vi "Lake Shore 335.vi"(6 "Setpoint":dbl format="%.4f", 7 "VISA resource name":refnum<visa-resource-name>, 8 "Range":u16(ring) items=["Off", "Low (On)", "Medium", "High"], 9 "Rate (D) (X.X %)":dbl=120.0 format="%.1f", 10 "Reset (I) (XX.X)":dbl=20.0 format="%.1f", 11 "Gain (P) (XX.X)":dbl=50.0 format="%.1f") -> (0 "Setpoint":dbl format="%.4f", 1 "Heater 1 (%)":dbl format="%.1f", 2 "Input B":dbl, 3 "Input A":dbl)   [LabVIEW 2012]
doc: "This example VI demonstrates the proper use of the Sensor Data (Multiple Readings) VI. This VI reads and returns multiple sensor readings from the instrument. Control over interval between readings is also provided."
uses:
  <instrlib>/Lake Shore 335/Public/Data/Sensor Data (Single Reading).vi
  <instrlib>/Lake Shore 335/Lake Shore 335.lvlib
panel:
  in  "Manual Output":dbl format="%.2f"
  out "Rate (D)":dbl format="%.1f"
  out "Reset (I)":dbl=20.0 format="%.1f"
  out "Gain (P)":dbl=50.0 format="%.1f"
  in  "Unit":u16(ring)=1 items=["Kelvin", "Celcius", "Sensor"]
  in  "Unit":u16(ring)=1 items=["Kelvin", "Celcius", "Sensor"]
  in  "stop":bool
  in  "Serial Configuration":T1={"Baud Rate"=57600, "Parity"=1, "Data Bits"=7, "Stop Bits"=10, "Flow Control"=0} {"Flow Control" items=["None", "XON/XOFF", "RTS/CTS", "XON/XOFF & RTS/CTS", "DTR/DSR", "XON/XOFF & DTR/DSR"]; "Stop Bits" items=["1.0"=10, "1.5"=15, "2.0"=20]; "Data Bits" items=["7"=7, "8"=8]; "Parity" items=["None", "Odd", "Even", "Mark", "Space"]; "Baud Rate" items=["300"=300, "600"=600, "1200"=1200, "2400"=2400, "4800"=4800, "9600"=9600, "19200"=19200, "38400"=38400, "57600"=57600]}
  # "Setpoint Configuration"
  # "Sensor Data"
  # "PID Configuration"
  # "Connection Settings"
  # "PID Controlling on Input A"
  # "PID Controlling on Input A"
  # "PID Read Oud (Check)"
  # "Heater Output"
  # "Setpoint Read Out (Check)"
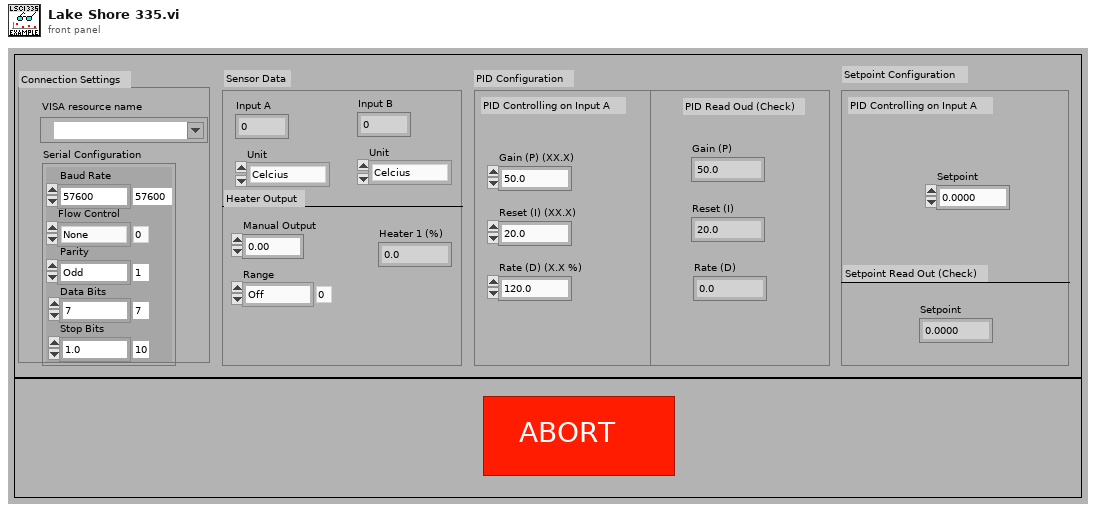
[diagram p1: front panel]
types:
  T1 = cluster{"Baud Rate":u32, "Parity":u16, "Data Bits":u16, "Stop Bits":u16, "Flow Control":u16}
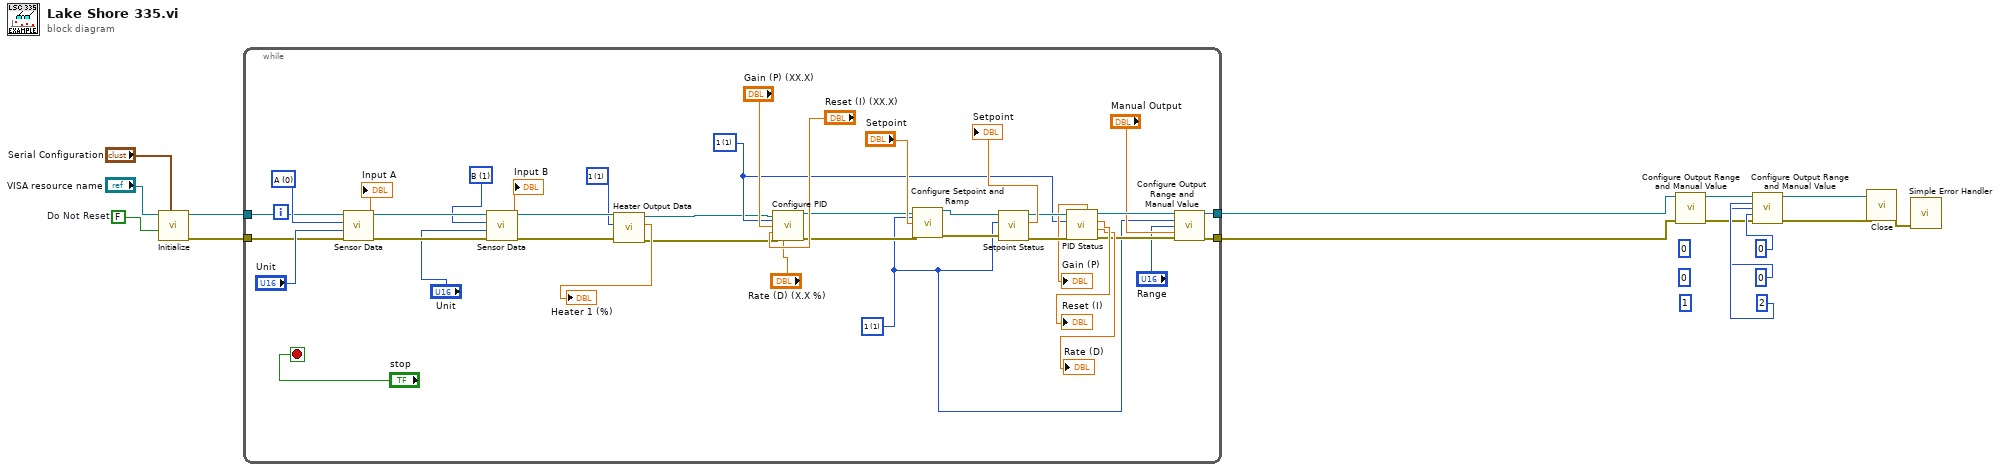
[diagram p0: block diagram]
diagram:
  (unwired) 1
  (unwired) 0
  (unwired) 0
  w14 = FALSE  # Do Not Reset
  n1 = call <instrlib>:"Initialize.vi"("Serial Configuration"="Serial Configuration", "Reset (True)"=w14, "VISA resource name"="VISA resource name") -> ("error out"=w11:errorcluster, "VISA resource name out"=w12:refnum<visa-resource-name>)  [unwired: 7 in]
  n2 = while {
    tunnel: w12 -> [w51]
    tunnel: w11 -> [w50]
    tunnel: [w27] -> w9
    tunnel: [w26] -> w8
    stop <- "stop" stop-if-true
    w19 = u16 1 items=["1"=1, "2"=2] ("Output's Control Loop (1:1)")
    w18 = u16 1 items=["1"=1, "2"=2] ("Output's Control Loop (1:1)")
    w42 = u16 1 items=["1"=1, "2"=2] ("Heater Output (1:1)")
    w46 = u16 1 items=["A", "B"] ("Input (0:A)")
    w52 = u16 0 items=["A", "B"] ("Input (0:A)")
    n3 = call-poly <instrlib>:"Sensor Data.vi"("error in (no error)"=w50, "Data Source (0:Kelvin)"="Unit", "Input (0:A)"=w52, "VISA resource name"=w51) -> ("error out"=w48:errorcluster, "Sensor Data"=→"Input A":dbl, "VISA resource name out"=w49:refnum<visa-resource-name>)  [unwired: 5 in]
    n4 = call-poly <instrlib>:"Sensor Data.vi"("error in (no error)"=w48, "Data Source (0:Kelvin)"="Unit", "Input (0:A)"=w46, "VISA resource name"=w49) -> ("error out"=w43:errorcluster, "Sensor Data"=→"Input B":dbl, "VISA resource name out"=w44:refnum<visa-resource-name>)  [unwired: 5 in]
    n5 = call <instrlib>:"Heater Output Data.vi"("error in (no error)"=w43, "Heater Output (1:1)"=w42, "VISA resource name"=w44) -> ("error out"=w16:errorcluster, "Output Value"=→"Heater 1 (%)":dbl, "VISA resource name out"=w17:refnum<visa-resource-name>)  [unwired: 6 in]
    n6 = call <instrlib>:"Configure PID.vi"("VISA resource name"=w17, "Output's Control Loop (1:1)"=w18, "Gain (P) (50.0)"="Gain (P) (XX.X)", "Reset (I) (20.0)"="Reset (I) (XX.X)", "error in (no error)"=w16, "Rate (D) (0.0 %)"="Rate (D) (X.X %)") -> ("VISA resource name out"=w21:refnum<visa-resource-name>, "error out"=w20:errorcluster)  [unwired: 8 in]
    n7 = call <instrlib>:"Configure Setpoint and Ramp.vi"("VISA resource name"=w21, "Output's Control Loop (1:1)"=w19, "Setpoint (0.0000)"="Setpoint", "error in (no error)"=w20) -> ("VISA resource name out"=w38:refnum<visa-resource-name>, "error out"=w37:errorcluster)  [unwired: 10 in]
    n8 = call <instrlib>:"Setpoint Status.vi"("error in (no error)"=w37, "Output (1:1)"=w19, "VISA resource name"=w38) -> ("error out"=w33:errorcluster, "Setpoint"=→"Setpoint":dbl, "VISA resource name out"=w34:refnum<visa-resource-name>)  [unwired: 6 in]
    n9 = call <instrlib>:"PID Status.vi"("error in (no error)"=w33, "Output's Control Loop (1:1)"=w18, "VISA resource name"=w34) -> ("error out"=w28:errorcluster, "Rate (D)"=→"Rate (D)":dbl, "Reset (I)"=→"Reset (I)":dbl, "VISA resource name out"=w29:refnum<visa-resource-name>, "Gain (P)"=→"Gain (P)":dbl)  [unwired: 4 in]
    n10 = call <instrlib>:"Configure Output Range and Manual Value.vi"("VISA resource name"=w29, "Heater Output (1:1)"=w19, "Range (0:Off)"="Range", "Manual Output (0.00 %)"="Manual Output", "error in (no error)"=w28) -> ("VISA resource name out"=w27:refnum<visa-resource-name>, "error out"=w26:errorcluster)  [unwired: 9 in]
  }
  n11 = call <instrlib>:"Configure Output Range and Manual Value.vi"("VISA resource name"=w9, "error in (no error)"=w8) -> ("VISA resource name out"=w4:refnum<visa-resource-name>, "error out"=w3:errorcluster)  [unwired: 12 in]
  n12 = call <instrlib>:"Configure Output Range and Manual Value.vi"("VISA resource name"=w4, "Heater Output (1:1)"=2, "Range (0:Off)"=0, "Manual Output (0.00 %)"=0, "error in (no error)"=w3) -> ("VISA resource name out"=w2:refnum<visa-resource-name>, "error out"=w1:errorcluster)  [unwired: 9 in]
  n13 = call <instrlib>:"Close.vi"("error in (no error)"=w1, "VISA resource name"=w2) -> ("error out"=w10:errorcluster)  [unwired: 9 in]
  n14 = call <vilib>:"Simple Error Handler.vi"("error in (no error)"=w10) -> ()  [unwired: 4 in, 5 out]
